vi "Basic Receive.vi"() -> ()   [LabVIEW 2013, in "UART_Host_Driver.lvlib" / "UART Driver.lvclass"]
doc: "This example calls the UART Initialize, UART Configure Port, UART Execute Command, and a UART Close."
uses:
  UART Driver.lvclass
  Typedefs/Configuration Parameters.ctl
  FPGA/UART/StopBits.ctl
  FPGA/UART/Parity.ctl
  FPGA/UART/UART_Firmware.lvlib
  UART_Host_Driver.lvlib
panel:
  in  "Rx byte count":u32
  in  "Get Rx Data":bool
  out "Receive Data":string
  in  "stop":bool
  in  "Configuration Parameters":T1={"Baud"=115200, "Character Length"=8, "Stop Bits"=enum."1.0", "Parity"=enum."None", "Character Spacing (ticks)"=0}
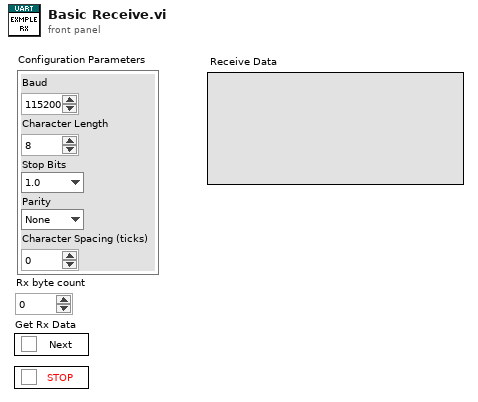
[diagram p1: front panel]
types:
  T1 = typedef "UART_Host_Driver.lvlib/Configuration Parameters.ctl" = cluster{"Baud":u32, "Character Length":u8, "Stop Bits":T2, "Parity":T3, "Character Spacing (ticks)":u32}
  T2 = typedef "UART_Firmware.lvlib/StopBits.ctl" = enum8{"1.0", "1.5", "2.0"}
  T3 = typedef "UART_Firmware.lvlib/Parity.ctl" = enum8{"None", "Even", "Odd"}
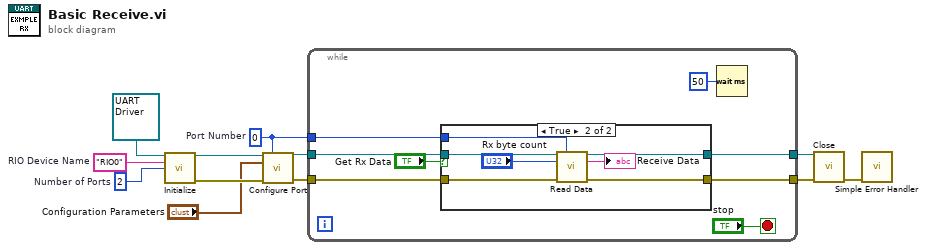
[diagram p0: block diagram]
diagram:
  w4 = u8 0  # Port Number
  w8 = u8 2  # Number of Ports
  w9 = "RIO0"  # RIO Device Name
  n1 = call-dynamic "Initialize.vi"("UART Driver in"=refnum<class "UART Driver.lvclass"> refnum, "RIO Device Name"=w9, "Number of UART Controllers"=w8) -> ("UART Driver out"=w12:refnum<class "UART Driver.lvclass">, "error out"=w11:errorcluster)  [unwired: 11 in]
  n2 = call-dynamic "Configure Port.vi"("UART Driver in"=w12, "Controller Number"=w4, "Configuration Parameters"="Configuration Parameters", "error in"=w11) -> ("UART Driver out"=w6:refnum<class "UART Driver.lvclass">, "error out"=w5:errorcluster)  [unwired: 10 in]
  n3 = while {
    tunnel: w6 -> [w20]
    tunnel: w5 -> [w19]
    tunnel: w4 -> [w18]
    tunnel: [w17] -> w3
    tunnel: [w16] -> w2
    stop <- "stop" stop-if-true
    n4 = case shown="True" "Get Rx Data" {
      tunnel: w20 -> [w22 w29]
      tunnel: w19 -> [w21 w28]
      tunnel: w18 -> [_ w27]
      tunnel: [w21 w26] -> w17
      tunnel: [w22 w25] -> w16
      frame False {
      }
      frame True {
        n5 = call-dynamic "Read Data.vi"("UART Driver in"=w29, "Port Number"=w27, "Rx byte count"="Rx byte count", "error in"=w28) -> ("UART Driver out"=w25:refnum<class "UART Driver.lvclass">, "Receive Data"=→"Receive Data":string, "error out"=w26:errorcluster)  [unwired: 9 in]
      }
    }
    n6 = Wait (ms)(milliseconds to wait=u32 50) -> ()  [unwired: 1 out]
  }
  n7 = call-dynamic "Close.vi"("UART Driver in"=w2, "error in"=w3) -> ("error out"=w1:errorcluster)  [unwired: 13 in]
  n8 = call <vilib>:"Simple Error Handler.vi"("error in (no error)"=w1) -> ()  [unwired: 4 in, 5 out]
